vi "ZoomDriveForward.vi"(8 "b Value":dbl=0.9 format="%#_13g", 9 "fastvalue":dbl=0.9 format="%#_13g", 10 "Mormal Value":dbl=0.8 format="%#_13g", 11 "Cluster In":T1={"Drive Forward Input "=0.0, "Drive Twist Input"=0.0, "Drive Output"=0.0, "Drivetwist Output"=0.0, "Left Joystick Buttons"=[FALSE, FALSE, FALSE, FALSE, FALSE, FALSE, FALSE, FALSE, FALSE, FALSE, FALSE, FALSE], "Left Joystick Axis"=[-0.007874015748031496, -0.0, -0.0, 0.18110236220472442], "Right Joystick Axis"=[], "Right Joystick Button"=[], "Arm Encoder"=4.0, "Left Drive Encoder"=0.0, "Right Drive Encoder"=1337462.0, "Gyro Angle "=188.0419921875, "Arm Joystick Output  "=0.0, "Line Follower L, C, R "=[TRUE, TRUE, TRUE], "Line follow?"=FALSE, " Climb Solenoid"=FALSE, "Wrist Encoder Count"=0.0, "Wrist Joystick Output"=0.0, "Ball Encoder Count"=0.0, "Ball Output"=0.0, "Climb Encoder"=0.0, "Climb Motor Output"=0.0, " Hatch Solenoid"=FALSE, "Arm Setpoint "=0.0, "Wrist Setpoint "=0.0, "Arm Joystick Enabled?"=FALSE, "Wrist Joystick Enabled"=FALSE, "Vision String"="", "Left Joystick POVs"=[-1]}) -> (3 "Cluster Out":T1={"Drive Forward Input "=0.0, "Drive Twist Input"=0.0, "Drive Output"=0.0, "Drivetwist Output"=0.0, "Left Joystick Buttons"=[FALSE, FALSE, FALSE, FALSE, FALSE, FALSE, FALSE, FALSE, FALSE, FALSE, FALSE, FALSE], "Left Joystick Axis"=[-0.007874015748031496, -0.0, -0.0, 0.18110236220472442], "Right Joystick Axis"=[], "Right Joystick Button"=[], "Arm Encoder"=4.0, "Left Drive Encoder"=0.0, "Right Drive Encoder"=1337462.0, "Gyro Angle "=188.0419921875, "Arm Joystick Output  "=0.0, "Line Follower L, C, R "=[TRUE, TRUE, TRUE], "Line follow?"=FALSE, " Climb Solenoid"=FALSE, "Wrist Encoder Count"=0.0, "Wrist Joystick Output"=0.0, "Ball Encoder Count"=0.0, "Ball Output"=0.0, "Climb Encoder"=0.0, "Climb Motor Output"=0.0, " Hatch Solenoid"=FALSE, "Arm Setpoint "=0.0, "Wrist Setpoint "=0.0, "Arm Joystick Enabled?"=FALSE, "Wrist Joystick Enabled"=FALSE, "Vision String"="", "Left Joystick POVs"=[-1]})   [LabVIEW 2018]
uses:
  TypeDefs/Teleop Data Cluster.ctl
  TypeDefs/Joystick Buttons.ctl
  TypeDefs/Joystick Axes.ctl
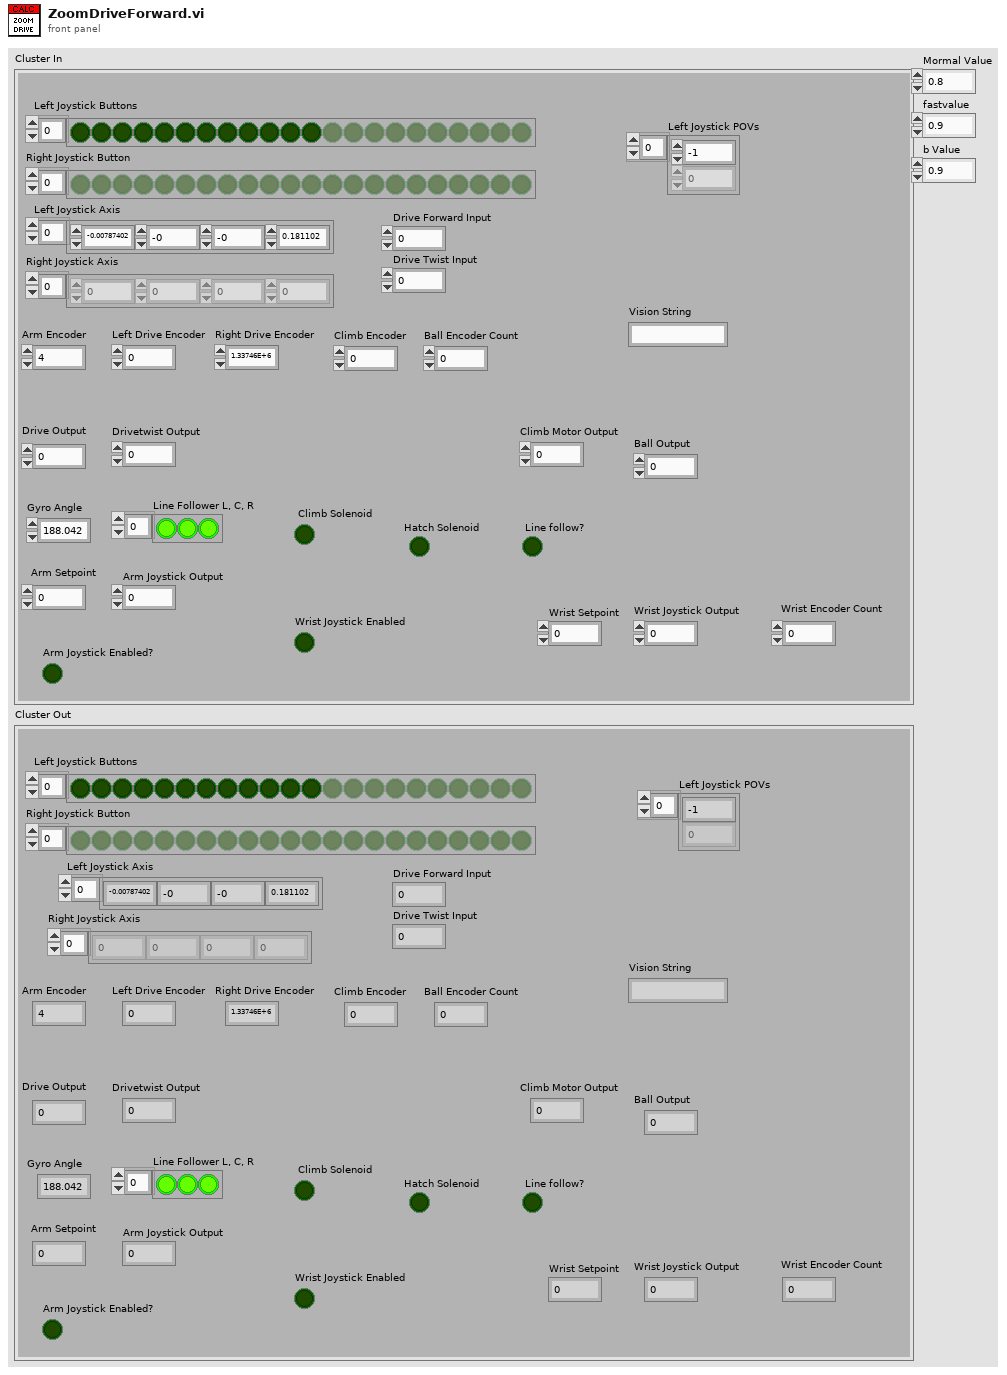
[diagram p1: front panel]
types:
  T1 = typedef "Teleop Data Cluster.ctl" = cluster{"Drive Forward Input ":dbl, "Drive Twist Input":dbl, "Drive Output":dbl, "Drivetwist Output":dbl, "Left Joystick Buttons":bool[], "Left Joystick Axis":dbl[], "Right Joystick Axis":dbl[], "Right Joystick Button":bool[], "Arm Encoder":dbl, "Left Drive Encoder":dbl, "Right Drive Encoder":dbl, "Gyro Angle ":dbl, "Arm Joystick Output  ":dbl, "Line Follower L, C, R ":bool[], "Line follow?":bool, " Climb Solenoid":bool, "Wrist Encoder Count":dbl, "Wrist Joystick Output":dbl, "Ball Encoder Count":dbl, "Ball Output":dbl, "Climb Encoder":dbl, "Climb Motor Output":dbl, " Hatch Solenoid":bool, "Arm Setpoint ":dbl, "Wrist Setpoint ":dbl, "Arm Joystick Enabled?":bool, "Wrist Joystick Enabled":bool, "Vision String":string, "Left Joystick POVs":i16[]}
  T2 = typedef "Joystick Axes.ctl" = enum16{"X Axis", "Y Axis", "Twist Axis", "Throttle"}
  T3 = typedef "Joystick Buttons.ctl" = enum16{"Trigger", "Thumb", "Top 3", "Top 4", "Top 5", "Top 6", "Bottom 7", "Bottom 8", "Bottom 9", "Bottom 10", "Bottom 11", "Bottom 12"}
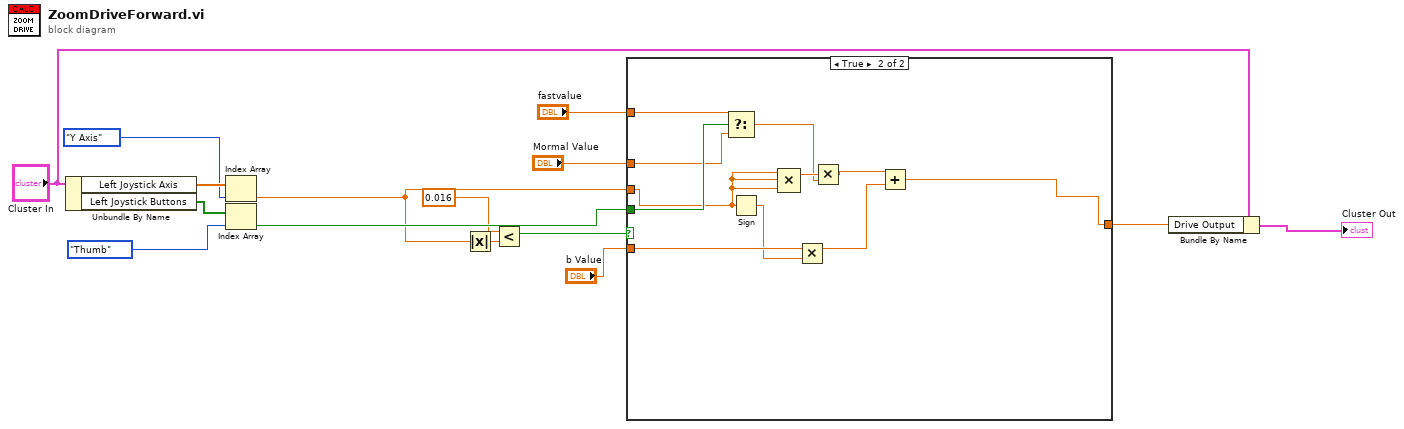
[diagram p0: block diagram]
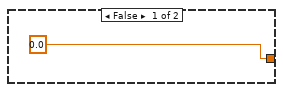
[diagram p2: hidden frame]
diagram:
  n1 = Unbundle By Name("Cluster In") -> ("Left Joystick Axis"=w15:dbl[], "Left Joystick Buttons"=w14:bool[])
  n2 = Index Array(array=w15, index=Joystick_Axes."Y Axis" ("Enum")) -> (element=w10:dbl)
  n3 = Index Array(array=w14, index=Joystick_Buttons."Thumb" ("Enum")) -> (element=w11:bool)
  n4 = Absolute Value(x=w10) -> (abs(x)=w9:dbl)
  n5 = Less?(x=0.016, y=w9) -> (x < y?=w7:bool)
  n6 = case shown="True" w7 {
    tunnel: w11 -> [_ w24]
    tunnel: w10 -> [_ w17]
    tunnel: [0.0 w27] -> w4
    tunnel: "Mormal Value" -> [_ w21]
    tunnel: "fastvalue" -> [_ w20]
    tunnel: "b Value" -> [_ w19]
    frame False {
    }
    frame True {
      n7 = Select(t=w20, s=w24, f=w21) -> (s? t:f=w23:dbl)
      n8 = Sign(1:w17) -> (0:w18:dbl)
      n9 = Compound Arithmetic op=MULTIPLY(w17, w17, w17) -> (w25:dbl)
      n10 = Multiply(x=w19, y=w18) -> (x*y=w22:dbl)
      n11 = Multiply(x=w25, y=w23) -> (x*y=w26:dbl)
      n12 = Add(x=w26, y=w22) -> (x+y=w27:dbl)
    }
  }
  n13 = Bundle By Name(cluster="Cluster In", "Drive Output"=w4) -> (→"Cluster Out":T1)
